vi "NanotecSMCPDDriver.set acceleration.vi"(0 "VISA resource name":refnum<visa-resource-name>, 1 "contollerID":i32=-1, 3 "acceleration [Hz/s]":i32, 5 "error in (no error)":errorcluster) -> (14 "VISA resource name out":refnum<visa-resource-name>, 15 "contollerID out":i32=-1, 19 "error out":errorcluster)   [LabVIEW 2014, in "NanotecSMCPDDriver.lvlib"]
doc: "Sets the acceleration that will be used for the trajectory of a movement."
uses:
  NanotecSMCPDDriver.lvlib
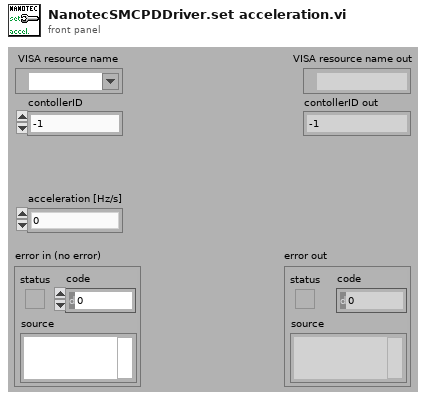
[diagram p1: front panel]
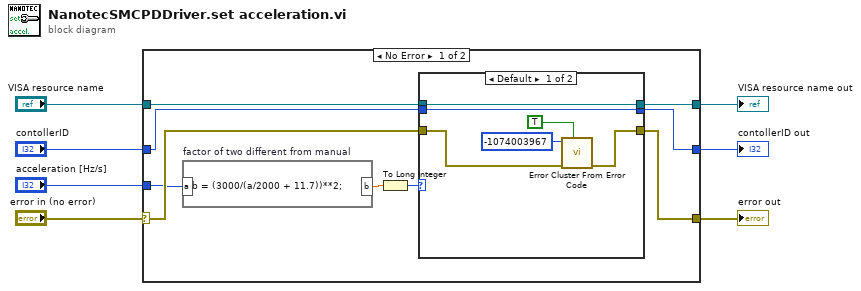
[diagram p0: block diagram]
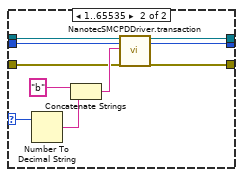
[diagram p2: hidden frame]
diagram:
  n1 = case shown="No Error" "error in (no error)" {
    selector: "error in (no error)" -> [w11 w33]
    tunnel: [w15 w35] -> w7
    tunnel: [w14 w33] -> w6
    tunnel: "VISA resource name" -> [w13 w35]
    tunnel: "contollerID" -> [w12 w34]
    tunnel: [w16 w34] -> w3
    tunnel: "acceleration [Hz/s]" -> [w10 _]
    frame No Error {
      n2 = formula code="b = (3000/(a/2000 + 11.7))**2;" "factor of two different from manual"("a"=w10) -> ("b"=w9:dbl)
      n3 = To Long Integer(number=w9) -> (32bit integer=w8:i32)
      n4 = case shown="Default" w8 {
        selector: w8 -> [_ w23]
        tunnel: [w18 w32] -> w16
        tunnel: [w19 w31] -> w15
        tunnel: [w22 w30] -> w14
        tunnel: w13 -> [w19 w26]
        tunnel: w12 -> [w18 w25]
        tunnel: w11 -> [w17 w24]
        frame Default {
          n5 = call <vilib>:"Error Cluster From Error Code.vi"("show call chain? (False)"=TRUE, "error in (no error)"=w17, "error code (0)"=-1074003967) -> ("error out"=w22:errorcluster)  [unwired: 6 in]
        }
        frame 1..65535 {
          n6 = Number To Decimal String(number=w23) -> (decimal integer string=w29:string)  [unwired: 1 in]
          n7 = Concatenate Strings("b" ("commandString"), w29) -> (w27:string)
          n8 = call "NanotecSMCPDDriver.transaction.vi"("VISAresource"=w26, "contollerID"=w25, "commandString"=w27, "error in (no error)"=w24) -> ("VISAresource out"=w31:refnum<visa-resource-name>, "contollerID out"=w32:i32, "error out"=w30:errorcluster)  [unwired: 10 in, 3 out]
        }
      }
    }
    frame Error {
    }
  }
  "VISA resource name out" <- w7
  "error out" <- w6
  "contollerID out" <- w3
